vi "SSL Detection Frame Simple Estimator Kalman.vi"(7 "Enable":bool, 8 "ignora esquerda?":bool=TRUE, 9 "ignora lado?":bool=TRUE, 10 "Field Size":T1, 11 "Detection Frame In":T2 {"robots_blue"."height" format="%+4.3f"; "robots_blue"."pixel_y" format="%+4.3f"; "robots_blue"."pixel_x" format="%+4.3f"; "robots_blue"."orientation" format="%+4.3f"; "robots_blue"."y" format="%+4.3f"; "robots_blue"."confidence" format="%4.3f"; "robots_blue"."x" format="%+4.3f"; "robots_yellow"."height" format="%+4.3f"; "robots_yellow"."pixel_y" format="%+4.3f"; "robots_yellow"."pixel_x" format="%+4.3f"; "robots_yellow"."orientation" format="%+4.3f"; "robots_yellow"."y" format="%+4.3f"; "robots_yellow"."confidence" format="%4.3f"; "robots_yellow"."x" format="%+4.3f"}) -> (2 "Field Size Out":T1, 3 "Detection Frame Out":T2 {"robots_blue"."height" format="%+4.3f"; "robots_blue"."pixel_y" format="%+4.3f"; "robots_blue"."pixel_x" format="%+4.3f"; "robots_blue"."orientation" format="%+4.3f"; "robots_blue"."y" format="%+4.3f"; "robots_blue"."confidence" format="%4.3f"; "robots_blue"."x" format="%+4.3f"; "robots_yellow"."height" format="%+4.3f"; "robots_yellow"."pixel_y" format="%+4.3f"; "robots_yellow"."pixel_x" format="%+4.3f"; "robots_yellow"."orientation" format="%+4.3f"; "robots_yellow"."y" format="%+4.3f"; "robots_yellow"."confidence" format="%4.3f"; "robots_yellow"."x" format="%+4.3f"})   [LabVIEW 2017]
uses:
  SSL Detection Robot.ctl
  SSL Detection Ball.ctl
  SSL Detection Frame.ctl
  <vilib>/Analysis/Matrix/Datatypes/RealMatrix.ctl
  <vilib>/Analysis/Matrix/NI_Matrix.lvlib
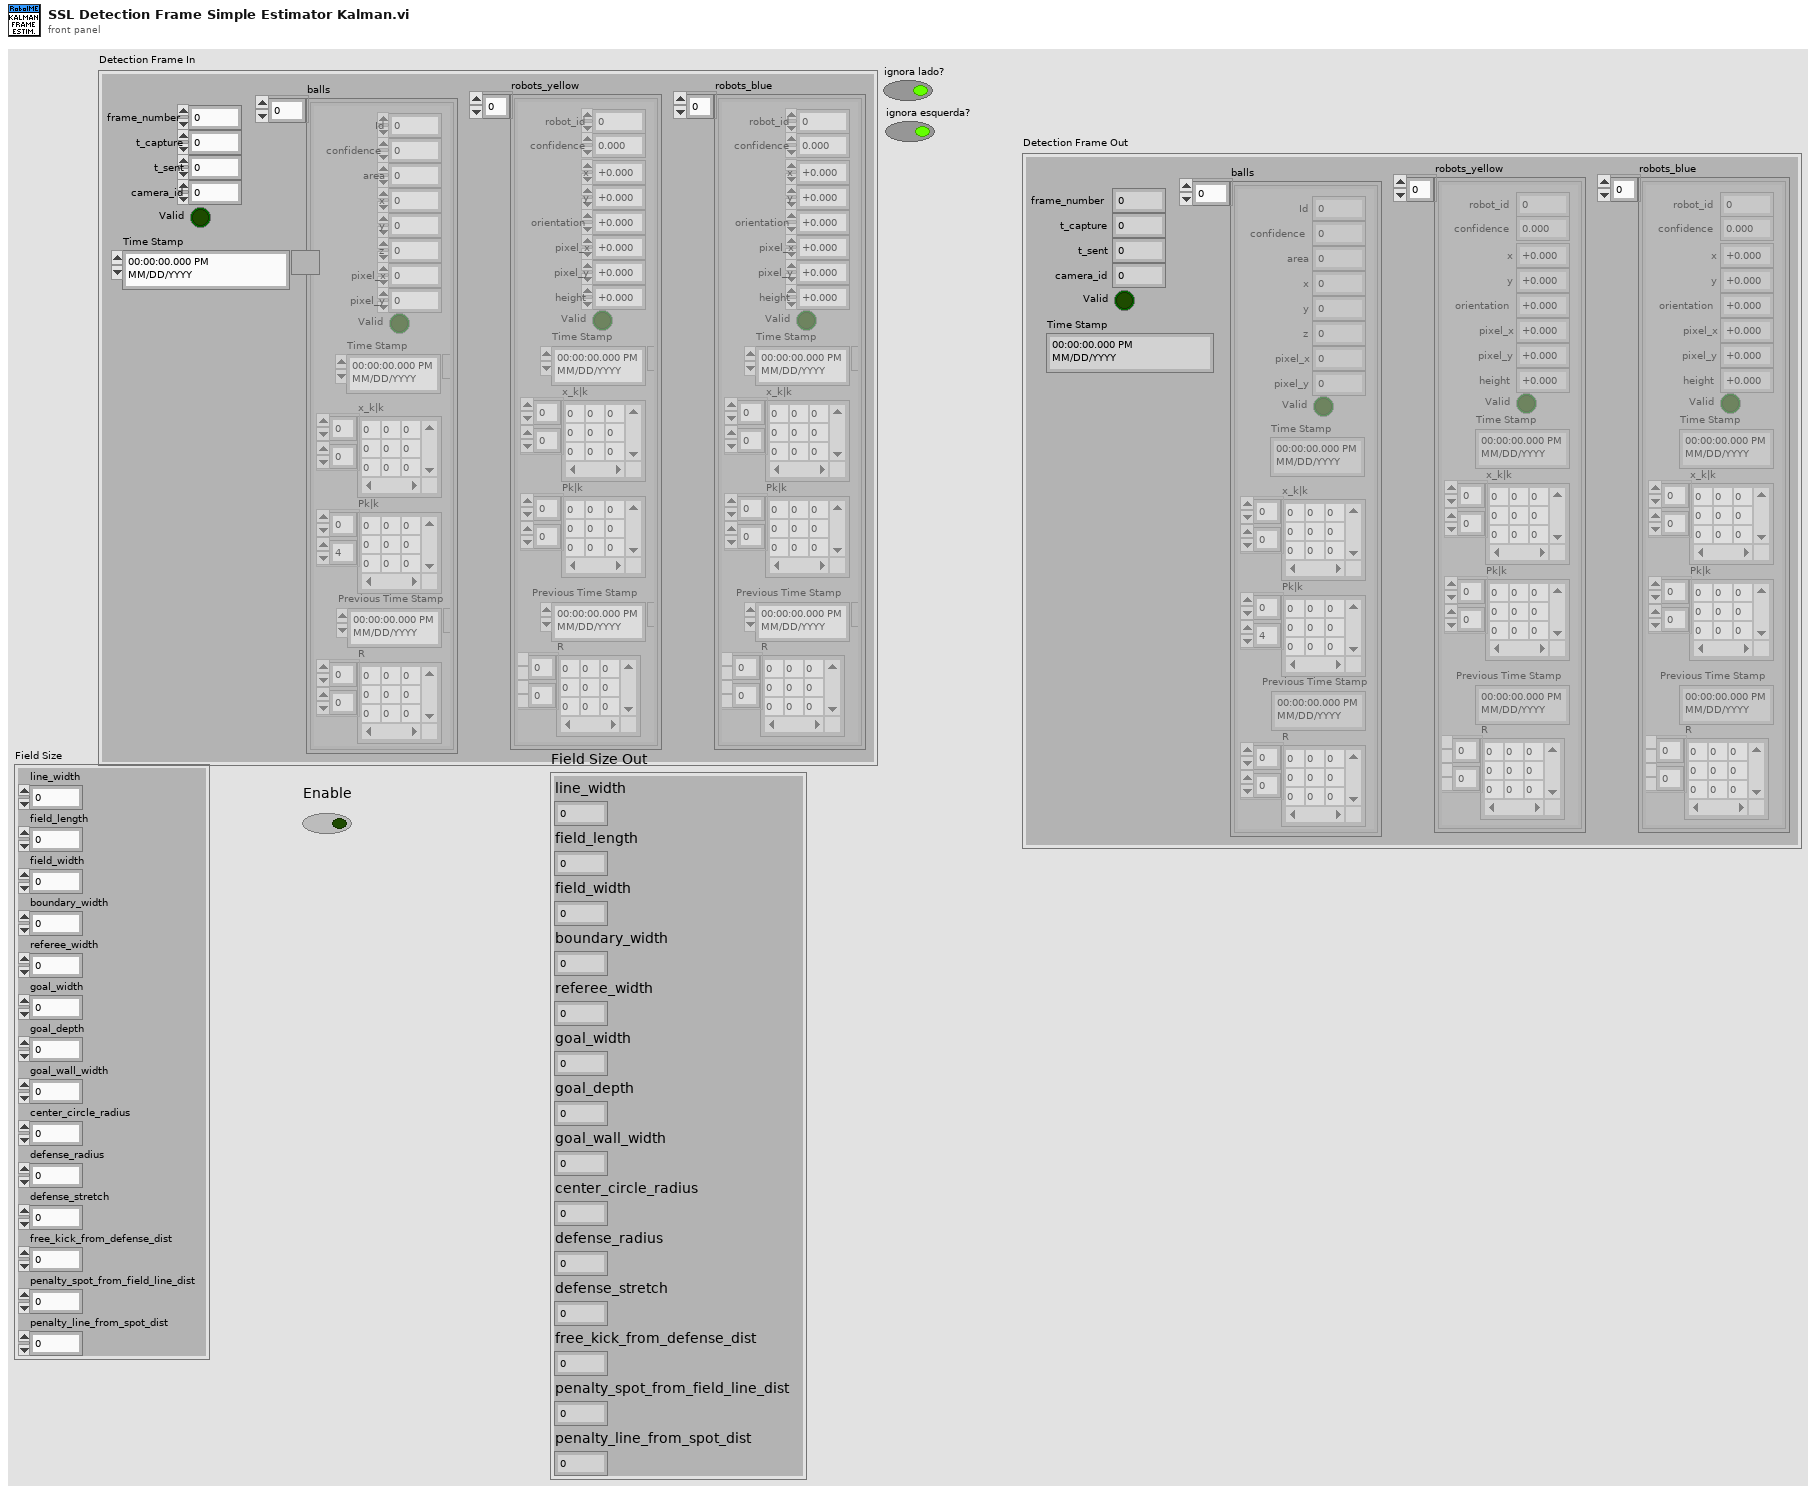
[diagram p1: front panel]
types:
  T1 = cluster{"line_width":u32, "field_length":u32, "field_width":u32, "boundary_width":u32, "referee_width":u32, "goal_width":u32, "goal_depth":u32, "goal_wall_width":u32, "center_circle_radius":u32, "defense_radius":u32, "defense_stretch":u32, "free_kick_from_defense_dist":u32, "penalty_spot_from_field_line_dist":u32, "penalty_line_from_spot_dist":u32}
  T2 = typedef "SSL Detection Frame.ctl" = cluster{"frame_number":u32, "t_capture":dbl, "t_sent":dbl, "camera_id":u32, "robots_yellow":T3[], "robots_blue":T3[], "balls":T5[], "Valid":bool, "Time Stamp":timestamp}
  T3 = typedef "SSL Detection Robot.ctl" = cluster{"x":sgl, "robot_id":u32, "confidence":sgl, "y":sgl, "orientation":sgl, "pixel_x":sgl, "pixel_y":sgl, "height":sgl, "Valid":bool, "Time Stamp":timestamp, "x_k|k":T4, "Pk|k":T4, "Previous Time Stamp":timestamp, "R":T4}
  T4 = typedef "NI_Matrix.lvlib/RealMatrix.ctl" = dbl[][]
  T5 = typedef "SSL Detection Ball.ctl" = cluster{"x":sgl, "area":u32, "confidence":sgl, "y":sgl, "z":sgl, "pixel_x":sgl, "pixel_y":sgl, "Valid":bool, "Time Stamp":timestamp, "x_k|k":T4, "Pk|k":T4, "Id":u32, "Previous Time Stamp":timestamp, "R":T4}
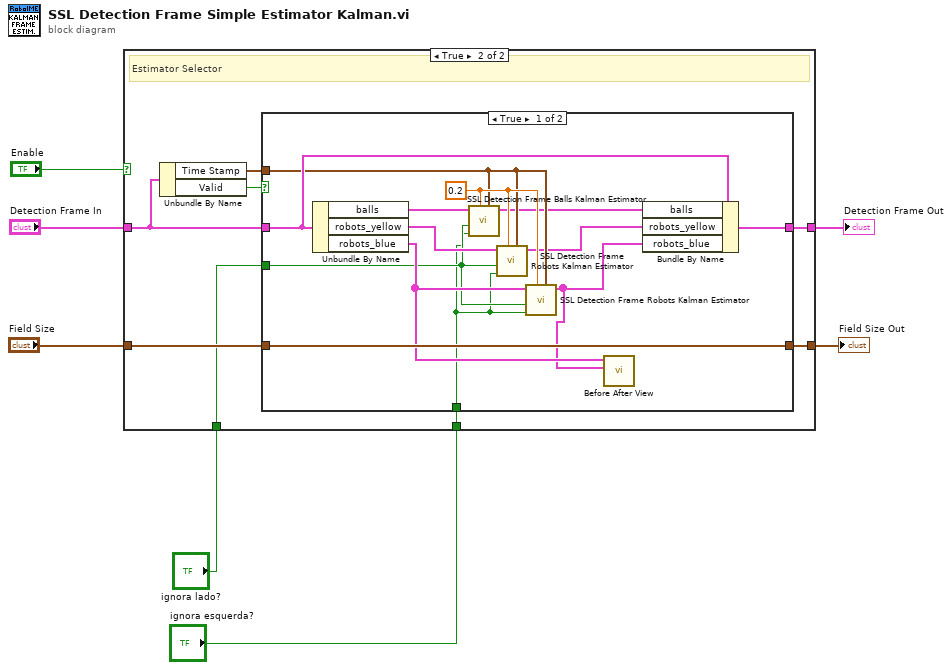
[diagram p0: block diagram]
diagram:
  n1 = case shown="True" "Enable" {
    tunnel: [w9 w17] -> w7
    tunnel: "Detection Frame In" -> [w9 w14]
    tunnel: "Field Size" -> [w8 w16]
    tunnel: [w8 w15] -> w4
    tunnel: "ignora lado?" -> [_ w11]
    tunnel: "ignora esquerda?" -> [_ w10]
    frame False {
    }
    frame True {
      # "Estimator Selector"
      n2 = Unbundle By Name(w14) -> ("Time Stamp"=w12:timestamp, "Valid"=w13:bool)
      n3 = case shown="True" w13 {
        tunnel: w14 -> [w30 w31]
        tunnel: [w29 w31] -> w17
        tunnel: w12 -> [w25 _]
        tunnel: w16 -> [w23 w32]
        tunnel: [w23 w32] -> w15
        tunnel: w11 -> [w19 _]
        tunnel: w10 -> [w18 _]
        frame True {
          w26 = 0.2 ("Life Time")
          n4 = Unbundle By Name(w30) -> ("balls"=w27:T5[], "robots_yellow"=w28:T3[], "robots_blue"=w22:T3[])
          n5 = call "SSL Detection Frame Balls Kalman Estimator.vi"("Time Stamp 2"=w25, "Life Time 2"=w26, "ignora esquerda?"=w18, "ignora lado"=w19, "Detection Ball \nArray"=w27) -> ("balls"=w20:T5[])  [unwired: 6 in]
          n6 = call "SSL Detection Frame Robots Kalman Estimator.vi"("Time Stamp"=w25, "Life Time"=w26, "ignora esquerda?"=w18, "ignora lado"=w19, "Robots"=w28) -> ("Robots Out"=w24:T3[])  [unwired: 6 in]
          n7 = call "SSL Detection Frame Robots Kalman Estimator.vi"("Time Stamp"=w25, "Life Time"=w26, "ignora esquerda?"=w18, "ignora lado"=w19, "Robots"=w22) -> ("Robots Out"=w21:T3[])  [unwired: 6 in]
          n8 = call "Before After View.vi"("after"=w21, "before"=w22) -> ()  [unwired: 10 in]
          n9 = Bundle By Name(cluster=w30, "balls"=w20, "robots_yellow"=w24, "robots_blue"=w21) -> (w29:T2)
        }
        frame False {
        }
      }
    }
  }
  "Detection Frame Out" <- w7
  "Field Size Out" <- w4
